vi "SwissSPAD Live_Refresh Single Parameter.vi"(7 "Verbose (T)":bool=TRUE, 8 "Error In":errorcluster, 9 "Data":variant, 10 "Control Label":string, 11 "VI Ref in":refnum<vi>) -> (0 "Error Out":errorcluster)   [LabVIEW 2021]
panel:
  out "Owning Tab Name":string
  out "Ctl found?":bool
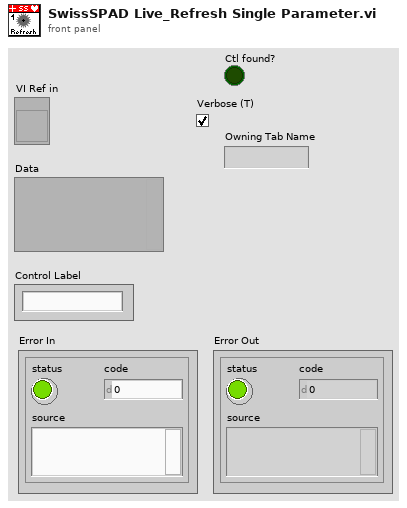
[diagram p1: front panel]
types:
  T1 = enum16{"Controls & Indicators", "Controls", "Indicators"}
  T2 = typedef "SwissSPAD Live_Settings List.ctl" = enum16{"FPGA:Bottom Half", "FPGA:Top Half", "FPGA:Bottom Bitfile Path", "FPGA:Top Bitfile Path", "FPGA:Bottom Bitstream Version", "FPGA:Top Bitstream Version", "FPGA:Auto Reset FPGA", "FPGA:Bottom FPGA Serial Number", "FPGA:Top FPGA Serial Number", "FPGA:Detector PCB Version", "Acquisition Parameters:Microlens", "Acquisition Parameters:SS2 DAQ Parameters", "Acquisition Parameters:Gate Configuration Array", "Acquisition Parameters:SS3 DAQ Parameters", "Acquisition Parameters:Buffer Size (# 8-bit Gates)", "File Information:File Information", "File Information:# Datasets in Series", "File Information:Scrambled File Flag", "File Information:SS3 Gate Slip Correction", "File Information:SS3 Hot Pixel Mismatch Detection", "File Information:Delay between Datasets", "File Information:Save Sum of All Gates Preview", "Image Parameters:Image ROI Information", "Image Parameters:Image Binning Options", "Image Parameters:SS3 Displayed Image", "Image Parameters:Image Display Options", "Image Parameters:Use Histogram Cursors", "Image Parameter:FPGA Data to Display", "UI Settings:Histogram Bins Number", "UI Settings:Use Image Display Options", "UI Settings:Verbose Settings", "UI Settings:Verbose Saving"}
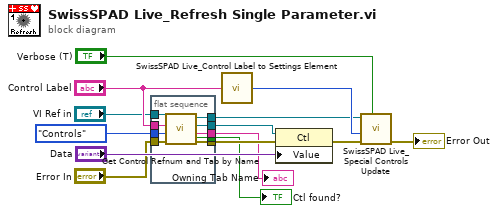
[diagram p0: block diagram]
diagram:
  n1 = flat-sequence {
    tunnel: "Control Label" -> [w23]
    tunnel: [w22] -> w12
    tunnel: [w21] -> w9
    tunnel: [w20] -> w8
    tunnel: T1."Controls" ("Selection") -> [w19]
    tunnel: "VI Ref in" -> [w18]
    tunnel: "Error In" -> [w17]
    tunnel: [w16] -> w2
    tunnel: [w15] -> w1
    frame #0 {
      n2 = call "Get Control Refnum and Tab by Name.vi"("error in"=w17, "Selection"=w19, "Control Label"=w23, "VI  Ref"=w18) -> ("error out"=w21:errorcluster, "Owning Tab Name"=w15:string, "Ctl Refnum"=w20:refnum<vi>, "VI  Ref (dup)"=w22:refnum<vi>, "Ctl found?"=w16:bool)  [unwired: 3 in]
    }
  }
  n3 = call "SwissSPAD Live_Control Label to Settings Element.vi"("Control Label"="Control Label") -> ("Settings List Element"=w14:T2)  [unwired: 8 in]
  n4 = property class="Ctl"(reference=w8, error in=w9, "Value"="Data") -> (error out=w11:errorcluster)  [unwired: 1 out]
  n5 = call "SwissSPAD Live_Special Controls Update.vi"("Verbose (T)"="Verbose (T)", "error in (no error)"=w11, "Settings List Element"=w14, "VI Refnum"=w12) -> ("Error Out"=→"Error Out":errorcluster)  [unwired: 7 in]
  "Ctl found?" <- w2
  "Owning Tab Name" <- w1
